vi "DelayGeneratorOpenSynchronization.vi"(9 "error in (no error)":errorcluster) -> (2 "Synchro":T1, 6 "error out":errorcluster)   [LabVIEW 2009]
uses:
  Controls/DelayGeneratorSynchro.ctl
  Controls/DelayGeneratorCommand.ctl
  Controls/DelayGeneratorState.ctl
  Controls/DelayTarget.ctl
  Aerotech/Controls/AerotechTarget.ctl
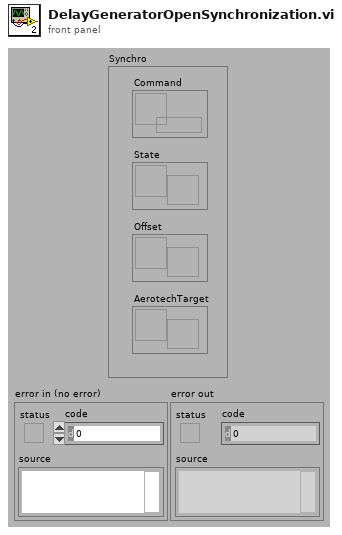
[diagram p1: front panel]
types:
  T1 = typedef "DelayGeneratorSynchro.ctl" = cluster{"Command":refnum<queue>, "State":refnum<notifier>, "Offset":refnum<notifier>, "AerotechTarget":refnum<notifier>}
  T2 = typedef "AerotechTarget.ctl" = cluster{"Time":timestamp, "Position":dbl, "Velocity":dbl}
  T3 = typedef "DelayGeneratorState.ctl" = enum16{"IDLING", "TRACKING", "STOPPING"}
  T4 = typedef "DelayTarget.ctl" = cluster{"Time":timestamp, "Position":dbl[unit], "Velocity":dbl[unit]}
  T5 = typedef "DelayGeneratorCommand.ctl" = enum16{"IDLE", "TRACK", "QUIT"}
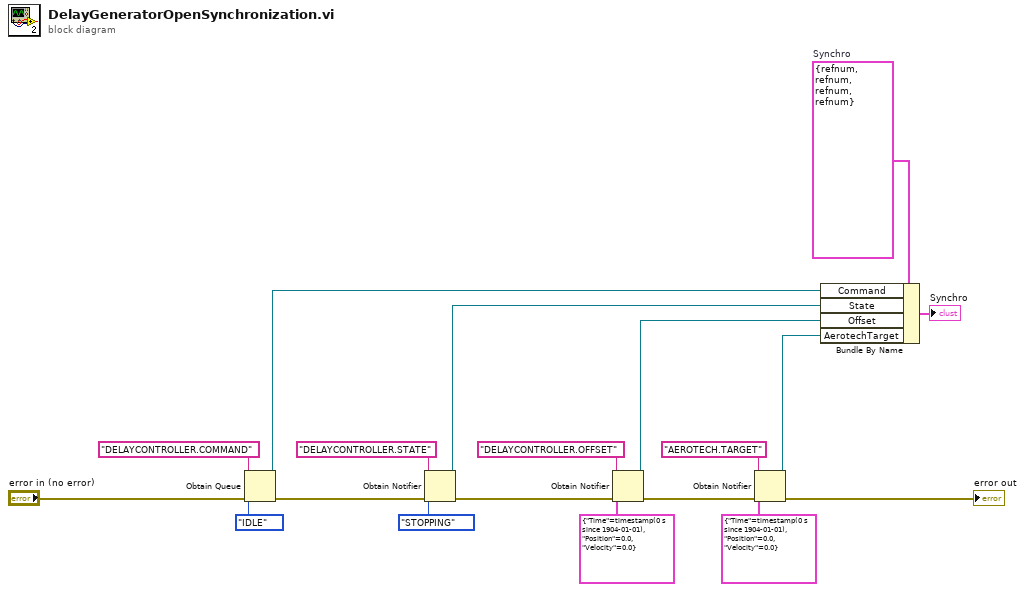
[diagram p0: block diagram]
diagram:
  w15 = T1 {"Command"=refnum, "State"=refnum, "Offset"=refnum, "AerotechTarget"=refnum}  # Synchro
  n1 = Obtain Queue(name (unnamed)="DELAYCONTROLLER.COMMAND", element data type=DelayGeneratorCommand."IDLE" ("DelayControllerCommand"), error in (no error)="error in (no error)") -> (queue out=w13:refnum<queue>, error out=w12:errorcluster)  [unwired: 2 in, 1 out]
  n2 = Obtain Notifier(name (unnamed)="DELAYCONTROLLER.STATE", notification data type=DelayGeneratorState."STOPPING" ("DelayGeneratorState")) -> (notifier out=w7:refnum<notifier>)  [unwired: 2 in, 2 out]
  n3 = Obtain Notifier(name (unnamed)="DELAYCONTROLLER.OFFSET", notification data type=T4 {"Time"=timestamp(0 s since 1904-01-01), "Position"=0.0, "Velocity"=0.0} ("DelayTarget"), error in (no error)=w12) -> (notifier out=w6:refnum<notifier>, error out=w3:errorcluster)  [unwired: 1 in, 1 out]
  n4 = Obtain Notifier(name (unnamed)="AEROTECH.TARGET", notification data type=T2 {"Time"=timestamp(0 s since 1904-01-01), "Position"=0.0, "Velocity"=0.0} ("AEROTECH.TARGET"), error in (no error)=w3) -> (notifier out=w1:refnum<notifier>, error out=→"error out":errorcluster)  [unwired: 1 in, 1 out]
  n5 = Bundle By Name(cluster=w15, "Command"=w13, "State"=w7, "Offset"=w6, "AerotechTarget"=w1) -> (→"Synchro":T1)
